vi "get top array index.vi"(8 "error in (no error)":errorcluster, 11 "Array in":refnum<vi>) -> (0 "error out":errorcluster, 2 "top index":u32, 3 "Array out":refnum<vi>)   [LabVIEW 2014, in "Tagbus PID Module editor node.lvclass"]
uses:
  Tagbus PID Module editor node.lvclass
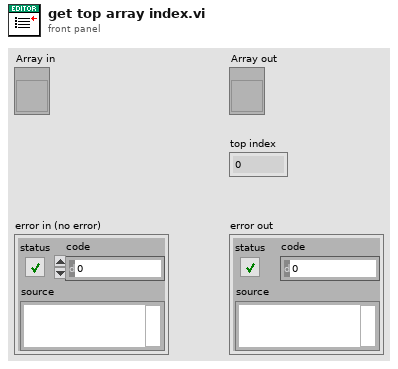
[diagram p1: front panel]
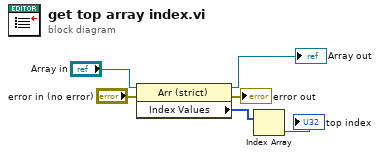
[diagram p0: block diagram]
diagram:
  n1 = property class="Arr (strict)"(reference="Array in", error in="error in (no error)") -> (reference out=→"Array out":refnum<vi>, error out=→"error out":errorcluster, "Index Values"=w6:u32[])
  n2 = Index Array(array=w6) -> (element=→"top index":u32)  [unwired: 1 in]
